vi "get_variable_start_values.vi"(8 "error in (no error)":errorcluster, 11 "Variable Settings":T1={"Measurements per Iteration"=1, "Local Data Path"=path "C:/Users/Saffmanlab/Documents/Cesium/data", "Experiment description suffix for filename (no spaces please)"="", "Network Data Path"=path "Z:/", "Copy data to network"=TRUE, "Measurement Timeout (ms)"=0, "Independent Variables"=[], "Dependent Variables"=[], "Run Test Mode"=FALSE} {"Independent Variables"."# steps" min=1 step=1; "Measurements per Iteration" min=1 step=1}) -> (0 "error out":errorcluster, 1 "dependent variable results":dbl[](array[numeric]), 2 "all variable names":string[](array[string]), 3 "all variable values (min or calculated)":dbl[](array[numeric]))   [LabVIEW 2012]
uses:
  ExperimentVariables/Variable_Settings.ctl
  ExperimentVariables/ExperimentVariables.lvclass
panel:
  # "Parameters will be evaluated once at the beginning of the experiment from top to bottom, \nso any parameter may depend on all those above it.\nVariables will be evaluated each iteration.\nParameters and Variables may be used in various other experiment settings, as noted.\nSee LabView Help -> Formula Node and Expression Node Functions for a list of available functions."
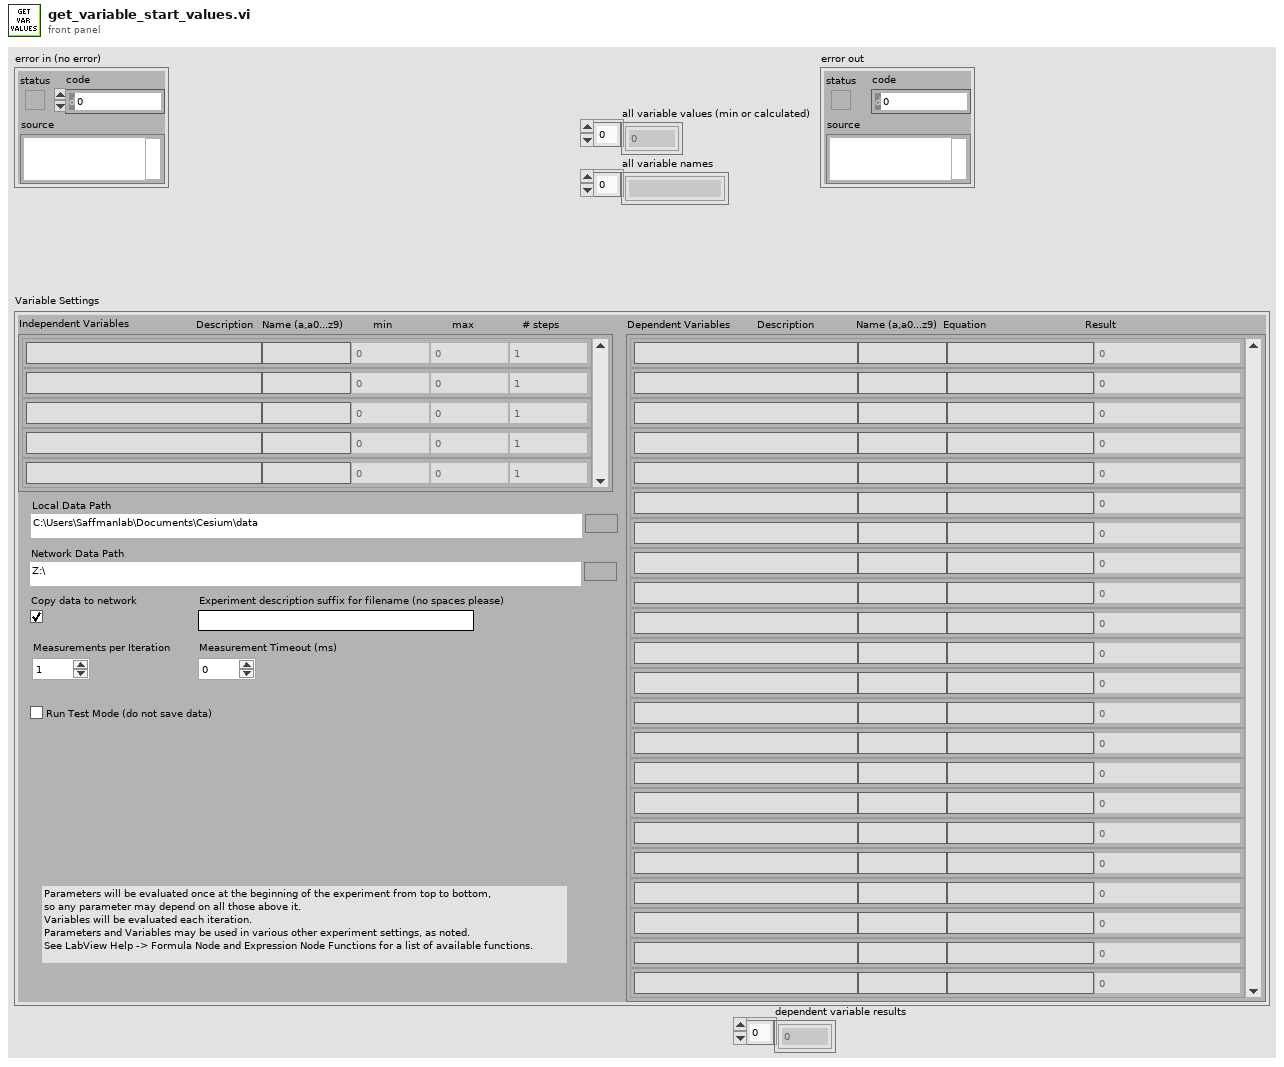
[diagram p1: front panel]
types:
  T1 = typedef "ExperimentVariables.lvclass/Variable_Settings.ctl" = cluster{"Measurements per Iteration":i32, "Local Data Path":path, "Experiment description suffix for filename (no spaces please)":string, "Network Data Path":path, "Copy data to network":bool, "Measurement Timeout (ms)":u32, "Independent Variables":cluster{"Description":string, "Name (a,a0...a9)":string, "min":dbl, "max":dbl, "# steps":u32}[], "Dependent Variables":cluster{"Description":string, "Name (a,a0...a9)":string, "Equation":string, "Result":dbl}[], "Run Test Mode":bool}
  T2 = cluster{"Description":string, "Name (a,a0...a9)":string, "min":dbl, "max":dbl, "# steps":u32}[]
  T3 = cluster{"Description":string, "Name (a,a0...a9)":string, "Equation":string, "Result":dbl}[]
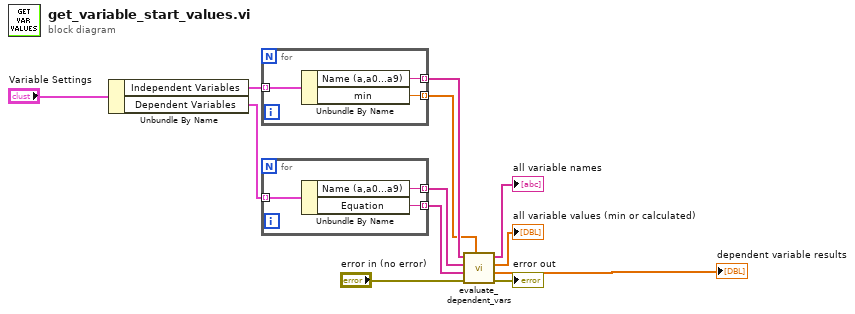
[diagram p0: block diagram]
diagram:
  n1 = Unbundle By Name("Variable Settings") -> ("Independent Variables"=w11:T2, "Dependent Variables"=w12:T3)
  n2 = for {
    tunnel: w11 -> [w15] mode=indexing
    tunnel: [w14] -> w7 mode=indexing
    tunnel: [w13] -> w6 mode=indexing
    n3 = Unbundle By Name(w15) -> ("Name (a,a0...a9)"=w14:string, "min"=w13:dbl)
  }
  n4 = for {
    tunnel: w12 -> [w18] mode=indexing
    tunnel: [w17] -> w8 mode=indexing
    tunnel: [w16] -> w9 mode=indexing
    n5 = Unbundle By Name(w18) -> ("Name (a,a0...a9)"=w17:string, "Equation"=w16:string)
  }
  n6 = call "evaluate_dependent_vars.vi"("current independent variable values"=w6, "error in (no error)"="error in (no error)", "dependent variable equations"=w9, "dependent variable names"=w8, "independent variable names"=w7) -> ("error out"=→"error out":errorcluster, "dependent variable results"=→"dependent variable results":dbl[], "current all variable values"=→"all variable values (min or calculated)":dbl[], "all variable names"=→"all variable names":string[])  [unwired: 3 in]
